vi "Test vib3.vi"() -> ()   [LabVIEW 2018]
uses:
  <vilib>/DAQmx/write.llb/DAQmx Write (Analog 1D DBL 1Chan NSamp).vi
  <vilib>/DAQmx/create/channels.llb/DAQmx Create Channel (AO-Voltage-Basic).vi
  <vilib>/DAQmx/configure/timing.llb/DAQmx Timing (Sample Clock).vi
  <vilib>/DAQmx/miscellaneous.llb/DAQmx Fill In Error Info.vi
  <resource>/objmgr/daqmx.rc
panel:
  in  "rate":dbl=1000.0 format="%0.2f"
  in  "physical channels":tag
  in  "source":tag
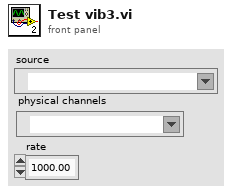
[diagram p1: front panel]
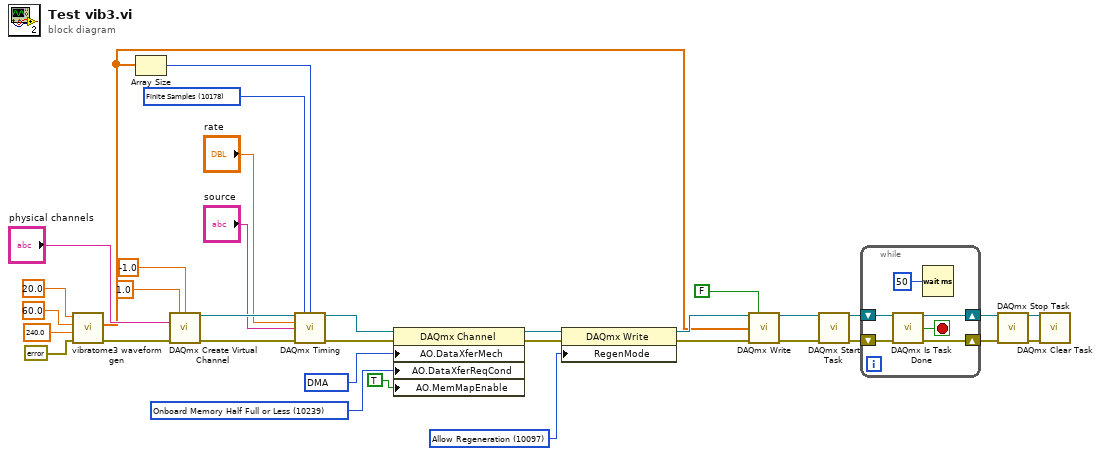
[diagram p0: block diagram]
diagram:
  w31 = 10178 items=["Finite Samples"=10178, "Continuous Samples"=10123, "Hardware Timed Single Point"=12522] ("sample mode")
  w26 = 10097 items=["Allow Regeneration"=10097, "Do Not Allow Regeneration"=10158] ("RegenMode")
  w29 = 10239 items=["Onboard Memory Empty"=10235, "Onboard Memory Half Full or Less"=10239, "Onboard Memory Less than Full"=10242] ("AO.DataXferReqCond")
  w30 = 10054 items=["DMA"=10054, "Interrupts"=10204, "Programmed I/O"=10264, "USB Bulk"=12590] ("AO.DataXferMech")
  n1 = call "vibratome3 waveform gen.vi"("error in"=errorcluster {"status"=FALSE, "code"=0, "source"=""}, "frequency(HZ)"=240.0, "slice time"=60.0, "ramp time(s)"=20.0) -> ("error out"=w1:errorcluster, "vib wave"=w5:dbl[])  [unwired: 6 in]
  n2 = Array Size(array=w5) -> (size(s)=w4:i32)
  n3 = call-poly <vilib>:"DAQmx Create Virtual Channel.vi"("maximum value"=1.0, "minimum value"=-1.0, "physical channels"="physical channels", "error in"=w1) -> ("task out"=w33:refnum<k21>, "error out"=w32:errorcluster)  [unwired: 10 in]
  n4 = call-poly <vilib>:"DAQmx Timing.vi"("task/channels in"=w33, "sample mode"=w31, "samples per channel"=w4, "rate"="rate", "source"="source", "error in"=w32) -> ("task out"=w21:refnum<k21>, "error out"=w22:errorcluster)  [unwired: 8 in]
  n5 = property class="DAQmx Channel"(reference=w21, error in=w22, "AO.DataXferMech"=w30, "AO.DataXferReqCond"=w29, "AO.MemMapEnable"=TRUE) -> (reference out=w27:refnum<k21>, error out=w3:errorcluster)
  n6 = property class="DAQmx Write"(reference=w27, error in=w3, "RegenMode"=w26) -> (reference out=w17:refnum<k21>, error out=w18:errorcluster)
  n7 = call-poly <vilib>:"DAQmx Write.vi"("task/channels in"=w17, "auto start"=FALSE, "data"=w5, "error in"=w18) -> ("task out"=w15:refnum<k21>, "error out"=w16:errorcluster)  [unwired: 9 in, 1 out]
  n8 = call <vilib>:"DAQmx Start Task.vi"("task/channels in"=w15, "error in"=w16) -> ("task out"=w11:refnum<k21>, "error out"=w12:errorcluster)  [unwired: 12 in]
  n9 = while {
    shift-right: [w38] -> w10
    shift-left: w11 -> [w37]
    shift-right: [w39] -> w9
    shift-left: w12 -> [w36]
    stop <- w40 stop-if-true
    n10 = call <vilib>:"DAQmx Is Task Done.vi"("task/channels in"=w37, "error in"=w36) -> ("task out"=w38:refnum<k21>, "task done?"=w40:bool, "error out"=w39:errorcluster)  [unwired: 11 in]
    n11 = Wait (ms)(milliseconds to wait=u32 50) -> ()  [unwired: 1 out]
  }
  n12 = call <vilib>:"DAQmx Stop Task.vi"("task/channels in"=w10, "error in"=w9) -> ("task out"=w13:refnum<k21>, "error out"=w14:errorcluster)  [unwired: 12 in]
  n13 = call <vilib>:"DAQmx Clear Task.vi"("task in"=w13, "error in"=w14) -> ()  [unwired: 13 in, 1 out]
